vi "SVFA FFT Spectrum (Real-Im) (N Ch).vi"(0 "scaled signals [EU]":waveform(dbl)[](array[waveform]), 2 "window":T1=1 items=["None"=0, "Hanning"=1, "Hamming"=2, "Blackman-Harris"=3, "Exact Blackman"=4, "Blackman"=5, "Flat Top"=6, "4 Term B-Harris "=7, "7 Term B-Harris"=8, "Low Sidelobe"=9, "Force"=64, "Exponential"=65, "Blackman Nuttall"=11, "Triangle"=30, "Bartlett-Hanning"=31, "Bohman"=32, "Parzen"=33, "Welch"=34, "Kaiser"=60, "Dolph-Chebyshev"=61, "Gaussian"=62], 5 "error in (no error)":errorcluster, 7 "averaging parameters":T9={"averaging mode"=enum."No averaging", "weighting mode"=enum."Exponential", "number of averages"=10, "linear mode"=enum."One shot"} {"number of averages" min=1 step=1}, 9 "restart averaging (F)":bool) -> (11 "averaging done":bool, 13 "averages completed":dbl, 14 "real parts [EU rms]":cluster{"f0":dbl, "df":dbl, "real part":dbl[]}[](array[cluster]) {"real part" format="%.2p"; "df" format="%.2p"; "f0" format="%.2p"}, 16 "imaginary parts [EU rms]":T8(array[cluster]) {"imaginary part" format="%.2p"; "df" format="%.2p"; "f0" format="%.2p"}, 17 "unit labels":string[](array[string]), 18 "spectrum info":T2[](array[typedef]) {"x-axis units" items=["Time (s)"=0, "Frequency-CB (Hz)"=1, "Frequency-CPB (Hz)"=1248, "Frequency-Arbitrary (Hz)"=2357, "Quefrency (s)"=2, "Revolutions (rev)"=3, "Order"=4, "Speed (RPM)"=11, "Speed (rad/s)"=21, "Index"=65535]; "weighting filter" items=["Linear", "A-weighting", "B-weighting", "C-weighting", "ITU-R 468-4", "Dolby", "CCITT", "C-message", "Wb", "Wc", "Wd", "We", "Wf", "Wh", "Wj", "Wk", "Wm", "AES17 20 kHz lowpass", "AES17 40 kHz lowpass", "AES17 20 kHz highpass", "AES17 40 kHz highpass"]; "dB reference [EU]" format="%.2f"; "engineering units" items=["custom..."=0, "V"=1, "A"=21, "C"=30, "pC"=31, "s"=32, "-"=29, "Pa"=2, "N"=20, "g"=3, "m/s^2"=4, "m/s"=5, "m"=6, "mm/s"=12, "mm"=13, "micron/s"=14, "micron"=15, "in/s^2"=7, "in/s"=8, "in"=9, "mil/s"=10, "mil"=11, "rad/s^2"=16, "rad/s"=17, "rad"=18, "deg/s^2"=26, "deg/s"=27, "deg"=28, "RPM"=22, "cycle/s^2"=23, "Hz"=24, "cycle"=25, "strain"=19]; "spectral info"."window" items=["None "=0, "Hanning"=1, "Hamming"=2, "Blackman-Harris"=3, "Exact Blackman"=4, "Blackman"=5, "Flat Top"=6, "4 Term B-Harris "=7, "7 Term B-Harris"=8, "Low Sidelobe"=9, "Force - Exponential"=10, "Gaussian"=62]}, 19 "error out":errorcluster)   [LabVIEW 2017]
doc: "Computes the Fast Fourier Transform (FFT) spectrum of <B>scaled signal [EU]</B>. This VI returns FFT results as the real and imaginary parts, or the first and second elements of the ordered pairs, of the FFT spectrum. Wire data to the <B>scaled signal [EU]</B> input to determine the polymorphic instance to use or manually select the instance."
uses:
  <vilib>/addons/_NISVFA/_Shared subVIs/Controls/svc_Spectrum Info.ctl
  <vilib>/addons/_NISVFA/_Shared subVIs/Controls/svc_X-Axis Units.ctl
  <vilib>/addons/_NISVFA/_Shared subVIs/Controls/svc_Spectrum Type.ctl
  <vilib>/addons/_NISVFA/_Shared subVIs/Controls/svc_Engineering Units Text Ring.ctl
  <vilib>/addons/_NISVFA/_Shared subVIs/Controls/svc_Weighting Filter Text Ring.ctl
  <vilib>/addons/_NISVFA/_Shared subVIs/Controls/svc_Complimentary Spectrum Units.ctl
  <vilib>/addons/_NISVFA/_Shared subVIs/Controls/svc_Window.ctl
  <vilib>/Analysis/2dsp.llb/Real FFT.vi
  <vilib>/Analysis/2dsp.llb/Power Spectrum (DBL).vi
  <vilib>/addons/_NISVFA/_Shared subVIs/Windowing/svfa_Scaled Time Domain Window (1 Ch).vi
  <vilib>/addons/_NISVFA/_Shared subVIs/Spectrum Info/svfa_Build Spectrum Info.vi
  <vilib>/addons/_NISVFA/_Shared subVIs/Spectrum Averaging/svfa_No Average Array (complex).vi
  <vilib>/addons/_NISVFA/_Shared subVIs/Spectrum Averaging/svfa_Average Array (complex).vi
  <vilib>/addons/_NISVFA/_Shared subVIs/Spectrum Averaging/svfa_No Average Array (real).vi
  <vilib>/addons/_NISVFA/_Shared subVIs/Spectrum Averaging/svfa_Average Array (real).vi
  <vilib>/addons/_NISVFA/_Shared subVIs/Spectrum Averaging/svfa_Peak Hold Array.vi
  <vilib>/addons/_NISVFA/_Shared subVIs/Windowing/svfa_Scaled Time Domain Window (Array).vi
  <vilib>/addons/_NISVFA/_Shared subVIs/Common/svc_Get SV Channel Info.vi
  <vilib>/addons/_NISVFA/_Shared subVIs/Common/svc_Spectrum Units.vi
  <vilib>/Analysis/4window.llb/Force Window.vi
  <vilib>/Analysis/4window.llb/Force Window (DBL).vi
  <vilib>/Analysis/4window.llb/Exponential Window.vi
  <vilib>/Analysis/4window.llb/Exponential Window (DBL).vi
  <vilib>/Utility/error.llb/Error Cluster From Error Code.vi
  <vilib>/Analysis/0measdsp.llb/Scaled Time Domain Window.vi
  <vilib>/Analysis/0measdsp.llb/Scaled Time Domain Window (DBL).vi
  <vilib>/addons/_NISVFA/_Spectrum Processing/subVIs/svfa_Spectrum Info Window to windowTd Type Def.vi
  <vilib>/addons/_NISVFA/_Shared subVIs/Common/svc_Window Parameters.vi
  <vilib>/addons/_NISVFA/_Shared subVIs/Common/svc_Get Window Info.vi
  <vilib>/addons/_NISVFA/_Shared subVIs/Common/svc_Get Weighting Enum and Labels.vi
  <vilib>/addons/_NISVFA/_Shared subVIs/Common/svc_Unit Label Lexical Class.vi
  <vilib>/addons/_NISVFA/_Shared subVIs/Common/svc_Engineering Units to Unit Label.vi
  <vilib>/addons/_NISVFA/_Shared subVIs/Common/svc_Format Value (DBL).vi
  <vilib>/addons/_NISVFA/_Shared subVIs/Common/svc_Channel Info to Spectrum Info.vi
  <vilib>/addons/_NISVFA/_Shared subVIs/Common/svc_Unit Label to Engineering Units.vi
  <vilib>/Analysis/NI_AALPro.lvlib
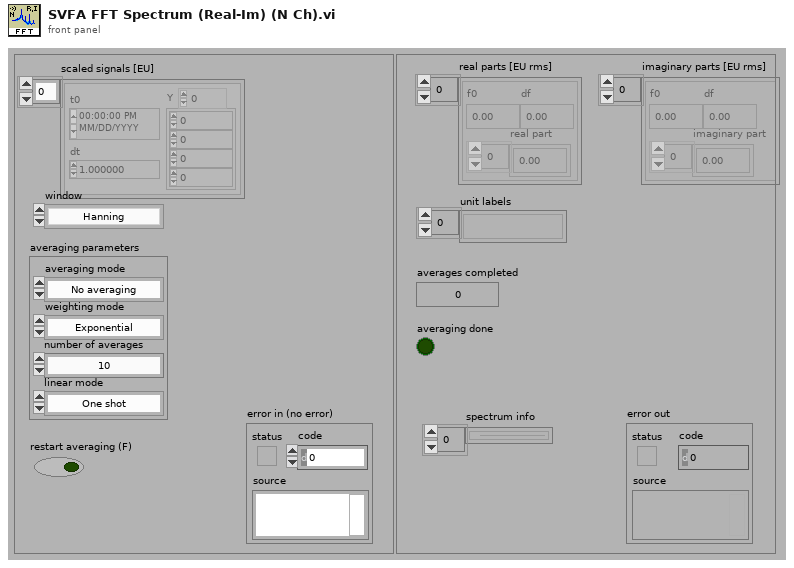
[diagram p1: front panel]
types:
  T1 = typedef "svc_Window.ctl" = u32
  T2 = typedef "svc_Spectrum Info.ctl" = cluster{"channel name":string, "description":string, "x-axis units":T3, "spectral info":cluster{"spectrum type":T4, "linear/dB":enum16{"linear", "dB"}, "window":u16, "window size":i32, "FFT size":i32}, "engineering units":T5, "custom label":string, "dB reference [EU]":dbl, "peak units":enum16{"rms", "peak", "peak-peak"}, "weighting filter":T6, "spectral density?":bool, "unit label":string, "spectrum skewed?":bool, "complimentary spectrum units":T7}
  T3 = typedef "svc_X-Axis Units.ctl" = u16
  T4 = typedef "svc_Spectrum Type.ctl" = enum16{"FFT Spectrum [complex]", "Amplitude [Magnitude]", "Power [Magnitude^2]", "Cross Spectrum [complex]", "Frequency Response [Complex]"}
  T5 = typedef "svc_Engineering Units Text Ring.ctl" = u16
  T6 = typedef "svc_Weighting Filter Text Ring.ctl" = u16
  T7 = typedef "svc_Complimentary Spectrum Units.ctl" = enum16{"none", "radians", "degrees", "cycles", "imaginary"}
  T8 = cluster{"f0":dbl, "df":dbl, "imaginary part":dbl[]}[]
  T9 = cluster{"averaging mode":enum16{"No averaging", "Vector averaging", "RMS averaging", "Peak hold"}, "weighting mode":enum16{"Linear", "Exponential"}, "number of averages":u32, "linear mode":enum16{"One shot", "Auto restart"}}
  T10 = cluster{"f0":dbl, "df":dbl, "complex spectrum":cdb[]}
  T11 = enum16{"Restart processing", "Continue processing", "Skip processing"}
  T12 = cluster{"complex FFT":cdb[], "real FFT":dbl[], "f0":dbl, "df":dbl, "averages completed":dbl, "averaging parameters":cluster{"averaging mode":enum16{"No averaging", "Vector averaging", "RMS averaging", "Peak hold"}, "weighting mode":enum16{"Linear", "Exponential"}, "number of averages":u32, "linear mode":enum16{"One shot", "Auto restart"}}}[]
  T13 = enum16{"No averaging", "Vector averaging", "RMS averaging", "Peak hold"}
  T14 = cluster{"complex FFT":cdb[], "real FFT":dbl[], "f0":dbl, "df":dbl, "averages completed":dbl, "averaging parameters":cluster{"averaging mode":enum16{"No averaging", "Vector averaging", "RMS averaging", "Peak hold"}, "weighting mode":enum16{"Linear", "Exponential"}, "number of averages":u32, "linear mode":enum16{"One shot", "Auto restart"}}}
  T15 = cluster{"complex FFT":cdb[], "Mag/Real FFT":dbl[], "f0":dbl, "df":dbl, "averages completed":dbl, "averaging parameters":cluster{"averaging mode":enum16{"No averaging", "Vector averaging", "RMS averaging", "Peak hold"}, "weighting mode":enum16{"Linear", "Exponential"}, "number of averages":u32, "linear mode":enum16{"One shot", "Auto restart"}}}
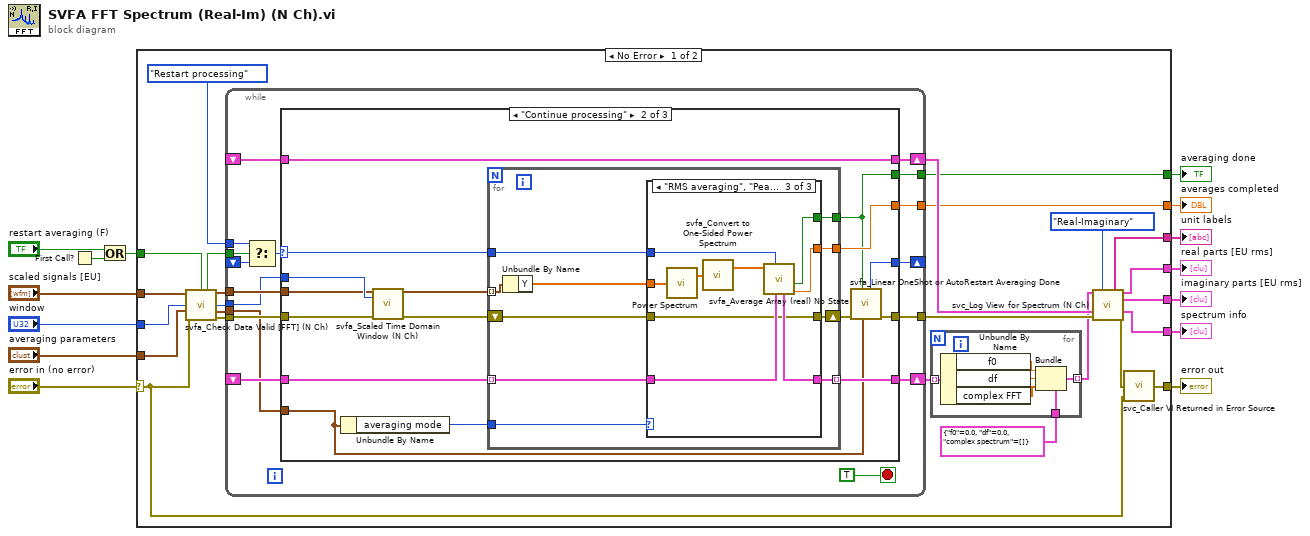
[diagram p0: block diagram]
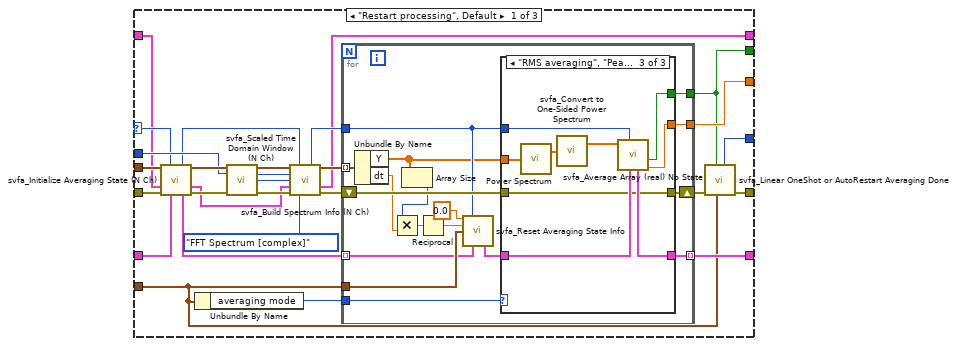
[diagram p2: hidden frame]
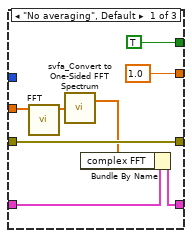
[diagram p3: hidden frame]
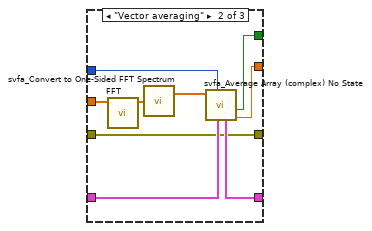
[diagram p4: hidden frame]
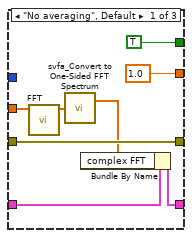
[diagram p5: hidden frame]
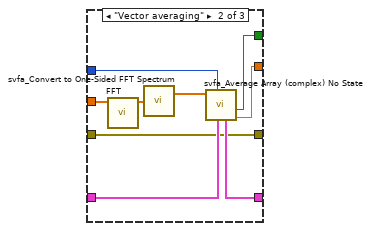
[diagram p6: hidden frame]
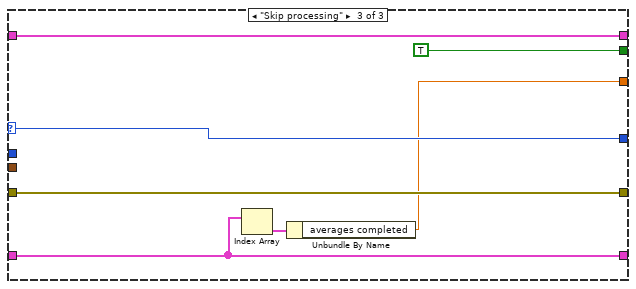
[diagram p7: hidden frame]
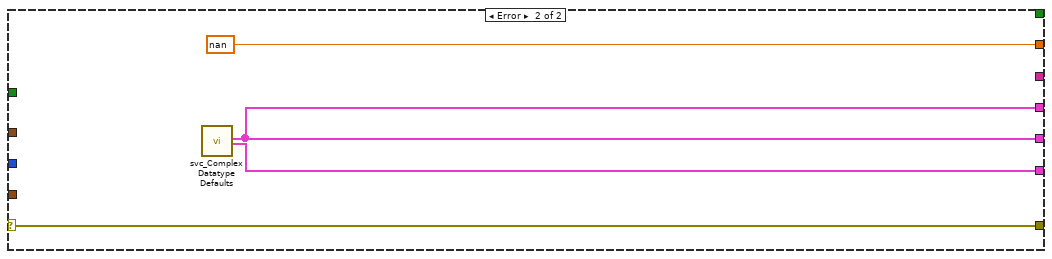
[diagram p8: hidden frame]
diagram:
  n1 = First Call?() -> (First Call?: T/F=w3:bool)
  n2 = Or(x="restart averaging (F)", y=w3) -> (x .or. y?=w1:bool)
  n3 = case shown="No Error" "error in (no error)" {
    selector: "error in (no error)" -> [w29 w195]
    tunnel: "scaled signals [EU]" -> [w39 _]
    tunnel: "averaging parameters" -> [w35 _]
    tunnel: w1 -> [w33 _]
    tunnel: [w30 w195] -> w11
    tunnel: [w38 w194] -> w10
    tunnel: [w19 _] -> w9
    tunnel: [w18 nan ("averages completed")] -> w8
    tunnel: [w36 w194] -> w7
    tunnel: [w32 _] -> w6
    tunnel: "window" -> [w34 _]
    tunnel: [w31 w193] -> w4
    frame No Error {
      n4 = call <vilib>:"svfa_Check Data Valid [FFT] (N Ch).vi"("scaled signals"=w39, "restart averaging (F)"=w33, "window"=w34, "averaging parameters"=w35, "error in (no error)"=w29) -> ("restart averaging"=w26:bool, "dup scaled signals"=w22:waveform(dbl)[], "dup window"=w23:T1, "dup averaging parameters"=w24:T9, "error out"=w25:errorcluster)  [unwired: 6 in]
      n5 = while {
        tunnel: [w60] -> w18
        tunnel: [w56] -> w19
        tunnel: [w54] -> w20
        shift-left: _ -> [w57]
        shift-right: [w58] -> w17
        tunnel: w25 -> [w59]
        tunnel: w22 -> [w61]
        shift-right: [w52] -> w21
        shift-left: _ -> [w53]
        tunnel: w23 -> [w51]
        tunnel: w24 -> [w50]
        tunnel: T11."Restart processing" ("t") -> [w49]
        tunnel: w26 -> [w48]
        shift-right: [w55] -> _
        shift-left: _ -> [w47]
        stop <- TRUE stop-if-true
        n6 = Select(t=w49, s=w48, f=w47) -> (s? t:f=w46:T11)
        n7 = case shown="\"Continue processing\"" w46 {
          selector: w46 -> [w78 w137 w192]
          tunnel: w61 -> [w90 w140 _]
          tunnel: [w88 w149 w188] -> w60
          tunnel: w59 -> [w69 w141 w191]
          tunnel: w51 -> [w85 w148 _]
          tunnel: w50 -> [w63 w134 _]
          tunnel: [w84 w147 w189] -> w58
          tunnel: w57 -> [w83 w138 w189]
          tunnel: [w82 w146 TRUE ("averaging done")] -> w56
          tunnel: [w81 w145 w192] -> w55
          tunnel: [w79 w143 w191] -> w54
          tunnel: w53 -> [w68 w139 w186]
          tunnel: [w66 w139 w186] -> w52
          frame "Restart processing", Default {
            n8 = call <vilib>:"svfa_Initialize Averaging State (N Ch).vi"("Windowed Waveform(s)"=w90, "processing control in"=w78, "spectra info in"=w68, "error in (no error)"=w69, "state info"=w83) -> ("processing control out"=w65:T11, "Windowed Waveform(s)"=w87:waveform(dbl)[], "spectra info out"=w67:T2[], "state info"=w89:T12, "error out"=w86:errorcluster)  [unwired: 6 in]
            n9 = Unbundle By Name(w63) -> ("averaging mode"=w70:T13)
            n10 = call <vilib>:"svfa_Scaled Time Domain Window (N Ch).vi"("Scaled signal(s)"=w87, "window"=w85, "error in (no error)"=w86) -> ("Windowed Waveform(s)"=w77:waveform(dbl)[], "window"=w76:T1, "window length"=w64:i32, "error out"=w75:errorcluster)  [unwired: 8 in, 1 out]
            n11 = call <vilib>:"svfa_Build Spectrum Info (N Ch).vi"("scaled signal(s)"=w77, "processing control in"=w65, "window"=w76, "window size"=w64, "spectra info in"=w67, "error in (no error)"=w75, "spectrum type"=svc_Spectrum_Type."FFT Spectrum [complex]") -> ("dup processing control"=w72:T11, "dup scaled signals"=w73:waveform(dbl)[], "spectra info out"=w66:T2[], "error out"=w74:errorcluster)  [unwired: 5 in]
            n12 = for {
              tunnel: w72 -> [w95]
              tunnel: w89 -> [w94] mode=indexing
              tunnel: [w104] -> w82
              tunnel: [w106] -> w88
              tunnel: w73 -> [w101] mode=indexing
              tunnel: w63 -> [w97]
              tunnel: [w105] -> w84 mode=indexing
              shift-right: [w107] -> w80
              shift-left: w74 -> [w102]
              tunnel: w70 -> [w103]
              n13 = Unbundle By Name ("Get Waveform Components")(w101) -> ("Y"=w92:dbl[], "dt"=w99:dbl)
              n14 = Array Size(array=w92) -> (size(s)=w91:i32)
              n15 = Multiply(x=w91, y=w99) -> (x*y=w100:dbl)
              n16 = Reciprocal(x=w100) -> (1/x=w96:dbl)
              n17 = call <vilib>:"svfa_Reset Averaging State Info.vi"("f0"=0.0, "processing control"=w95, "df"=w96, "averaging parameters"=w97, "averaging state info in"=w94) -> ("averaging state info out"=w93:T14)  [unwired: 9 in, 1 out]
              n18 = case shown="\"RMS averaging\", \"Peak hold\"" w103 {
                tunnel: w95 -> [_ w121 w130]
                tunnel: w93 -> [w112 w120 w129]
                tunnel: w92 -> [w109 w123 w132]
                tunnel: [w113 w116 w125] -> w107
                tunnel: [TRUE ("averaging done") w118 w126] -> w104
                tunnel: [1.0 ("averages completed") w117 w127] -> w106
                tunnel: w102 -> [w113 w116 w125]
                tunnel: [w111 w119 w128] -> w105
                frame "No averaging", Default {
                  n19 = call-poly <vilib>:"FFT.vi"("X"=w109) -> ("FFT {X}"=w110:cdb[])  [unwired: 9 in, 1 out]
                  n20 = call <vilib>:"svfa_Convert to One-Sided FFT Spectrum.vi"("two-sided FFT spectrum"=w110) -> ("one-sided FFT spectrum"=w108:cdb[])  [unwired: 1 out]
                  n21 = Bundle By Name(cluster=w112, "complex FFT"=w108) -> (w111:T14)
                }
                frame "Vector averaging" {
                  n22 = call-poly <vilib>:"FFT.vi"("X"=w123) -> ("FFT {X}"=w124:cdb[])  [unwired: 9 in, 1 out]
                  n23 = call <vilib>:"svfa_Convert to One-Sided FFT Spectrum.vi"("two-sided FFT spectrum"=w124) -> ("one-sided FFT spectrum"=w122:cdb[])  [unwired: 1 out]
                  n24 = call <vilib>:"svfa_Average Array (complex) No State.vi"("averaging state info in"=w120, "processing control"=w121, "array"=w122) -> ("averages completed"=w117:dbl, "averaging done"=w118:bool, "averaging state info out"=w119:T15)  [unwired: 5 in, 1 out]
                }
                frame "RMS averaging", "Peak hold" {
                  n25 = call-poly <vilib>:"Power Spectrum.vi"("X"=w132) -> ("Power Spectrum"=w133:dbl[])  [unwired: 1 out]
                  n26 = call <vilib>:"svfa_Convert to One-Sided Power Spectrum.vi"("two-sided power spectrum"=w133) -> ("one-sided power spectrum"=w131:dbl[])  [unwired: 1 out]
                  n27 = call <vilib>:"svfa_Average Array (real) No State.vi"("averaging state info in"=w129, "processing control"=w130, "array"=w131) -> ("averages completed"=w127:dbl, "averaging done"=w126:bool, "averaging state info out"=w128:T15)  [unwired: 5 in, 1 out]
                }
              }
            }
            n28 = call <vilib>:"svfa_Linear OneShot or AutoRestart Averaging Done.vi"("averaging parameters"=w63, "averaging done"=w82, "error in (no error)"=w80) -> ("error out"=w79:errorcluster, "processing control"=w81:T11)  [unwired: 7 in]
          }
          frame "Continue processing" {
            n29 = Unbundle By Name(w134) -> ("averaging mode"=w142:T13)
            n30 = call <vilib>:"svfa_Scaled Time Domain Window (N Ch).vi"("Scaled signal(s)"=w140, "window"=w148, "error in (no error)"=w141) -> ("Windowed Waveform(s)"=w135:waveform(dbl)[], "error out"=w136:errorcluster)  [unwired: 8 in, 3 out]
            n31 = for {
              tunnel: w137 -> [w151]
              tunnel: w138 -> [w150] mode=indexing
              tunnel: [w156] -> w146
              tunnel: [w158] -> w149
              tunnel: w135 -> [w153] mode=indexing
              tunnel: [w157] -> w147 mode=indexing
              shift-right: [w159] -> w144
              shift-left: w136 -> [w154]
              tunnel: w142 -> [w155]
              n32 = Unbundle By Name ("Get Waveform Components")(w153) -> ("Y"=w152:dbl[])
              n33 = case shown="\"RMS averaging\", \"Peak hold\"" w155 {
                tunnel: w151 -> [_ w173 w182]
                tunnel: w150 -> [w164 w172 w181]
                tunnel: w152 -> [w161 w175 w184]
                tunnel: [w165 w168 w177] -> w159
                tunnel: [TRUE ("averaging done") w170 w178] -> w156
                tunnel: [1.0 ("averages completed") w169 w179] -> w158
                tunnel: w154 -> [w165 w168 w177]
                tunnel: [w163 w171 w180] -> w157
                frame "No averaging", Default {
                  n34 = call-poly <vilib>:"FFT.vi"("X"=w161) -> ("FFT {X}"=w162:cdb[])  [unwired: 9 in, 1 out]
                  n35 = call <vilib>:"svfa_Convert to One-Sided FFT Spectrum.vi"("two-sided FFT spectrum"=w162) -> ("one-sided FFT spectrum"=w160:cdb[])  [unwired: 1 out]
                  n36 = Bundle By Name(cluster=w164, "complex FFT"=w160) -> (w163:T15)
                }
                frame "Vector averaging" {
                  n37 = call-poly <vilib>:"FFT.vi"("X"=w175) -> ("FFT {X}"=w176:cdb[])  [unwired: 9 in, 1 out]
                  n38 = call <vilib>:"svfa_Convert to One-Sided FFT Spectrum.vi"("two-sided FFT spectrum"=w176) -> ("one-sided FFT spectrum"=w174:cdb[])  [unwired: 1 out]
                  n39 = call <vilib>:"svfa_Average Array (complex) No State.vi"("averaging state info in"=w172, "processing control"=w173, "array"=w174) -> ("averages completed"=w169:dbl, "averaging done"=w170:bool, "averaging state info out"=w171:T15)  [unwired: 5 in, 1 out]
                }
                frame "RMS averaging", "Peak hold" {
                  n40 = call-poly <vilib>:"Power Spectrum.vi"("X"=w184) -> ("Power Spectrum"=w185:dbl[])  [unwired: 1 out]
                  n41 = call <vilib>:"svfa_Convert to One-Sided Power Spectrum.vi"("two-sided power spectrum"=w185) -> ("one-sided power spectrum"=w183:dbl[])  [unwired: 1 out]
                  n42 = call <vilib>:"svfa_Average Array (real) No State.vi"("averaging state info in"=w181, "processing control"=w182, "array"=w183) -> ("averages completed"=w179:dbl, "averaging done"=w178:bool, "averaging state info out"=w180:T15)  [unwired: 5 in, 1 out]
                }
              }
            }
            n43 = call <vilib>:"svfa_Linear OneShot or AutoRestart Averaging Done.vi"("averaging parameters"=w134, "averaging done"=w146, "error in (no error)"=w144) -> ("error out"=w143:errorcluster, "processing control"=w145:T11)  [unwired: 7 in]
          }
          frame "Skip processing" {
            n44 = Index Array(array=w189) -> (element=w187:T15)  [unwired: 1 in]
            n45 = Unbundle By Name(w187) -> ("averages completed"=w188:dbl)
          }
        }
      }
      n46 = for {
        tunnel: w17 -> [w45] mode=indexing
        tunnel: T10 {"f0"=0.0, "df"=0.0, "complex spectrum"=[]} ("cluster") -> [w44]
        tunnel: [w40] -> w15 mode=indexing
        n47 = Unbundle By Name(w45) -> ("f0"=w42:dbl, "df"=w43:dbl, "complex FFT"=w41:cdb[])
        n48 = Bundle(cluster=w44, "f0"=w42, "df"=w43, "complex spectrum"=w41) -> (w40:T10)
      }
      n49 = call <vilib>:"svc_Log View for Spectrum (N Ch).vi"("complex spectra"=w15, "View"=enum16{"Mag-Phase", "Real-Imaginary"}."Real-Imaginary", "spectra info in"=w21, "error in (no error)"=w20) -> ("unit label [mag or real]"=w32:string[], "magnitude or real"=w38:cluster{"f0":dbl, "df":dbl, "magnitude":dbl[]}[], "phase or imaginary"=w36:cluster{"f0":dbl, "df":dbl, "magnitude":dbl[]}[], "spectra info out"=w31:T2[], "error out"=w37:errorcluster)  [unwired: 6 in, 1 out]
      n50 = call <vilib>:"svc_Caller VI Returned in Error Source.vi"("warning input to caller"=w29, "error in (no error)"=w37) -> ("error out"=w30:errorcluster)  [unwired: 3 in]
    }
    frame Error {
      n51 = call <vilib>:"svc_Complex Datatype Defaults.vi"() -> ("empty array of spectra"=w194:cluster{"f0":dbl, "df":dbl, "magnitude":dbl[]}[], "empty array of spectrum info"=w193:T2[])  [unwired: 11 in, 7 out]
    }
  }
  "error out" <- w11
  "averaging done" <- w9
  "averages completed" <- w8
  "unit labels" <- w6
  "real parts [EU rms]" <- w10
  "imaginary parts [EU rms]" <- w7
  "spectrum info" <- w4
